vi "TestFGV.vi"() -> ()   [LabVIEW 2015]
uses:
  TypeDef/RoomsActionEnum.ctl
panel:
  out "Flag Out 4":bool[](array[boolean])
  out "Flag Out 3":bool[](array[boolean])
  out "Flag Out 2":bool[](array[boolean])
  out "Flag Out":bool[](array[boolean])
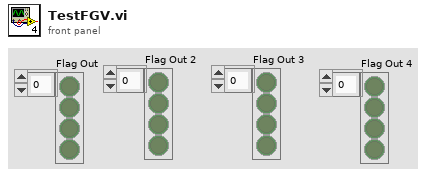
[diagram p1: front panel]
types:
  T1 = typedef "RoomsActionEnum.ctl" = enum16{"Init", "Add Room", "Remove Room", "Read Room", "Read Flag", "Read Flag State", "Write Flag State", "Read Flag Color", "Write Flag Color", "Read Bed Vacant", "Write Bed Vacant", "Read Personnel", "Add Personnel", "Remove Personnel", "Read Requests", "Add Request", "Remove Request", "Read Beacon ID", "Write Beacon ID", "Write Bed URL", "Read Bed URL"}
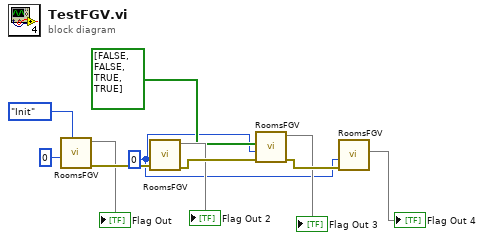
[diagram p0: block diagram]
diagram:
  w1 = 0 ("Room")
  n1 = call "RoomsFGV.vi"("Actions"=RoomsActionEnum."Init", "Data In"=0 ("Room")) -> ("error out"=w12:errorcluster, 2:→"Flag Out")  [unwired: 7 in, 1 out]
  n2 = call "RoomsFGV.vi"("error in (no error)"=w12, "Data In"=w1) -> ("error out"=w11:errorcluster, 2:→"Flag Out 2", "Actions"=w8:T1)  [unwired: 6 in, 1 out]
  n3 = call "RoomsFGV.vi"("error in (no error)"=w11, "Data In"=w1, "Room"=bool[] [FALSE, FALSE, TRUE, TRUE] ("Flag In")) -> ("error out"=w10:errorcluster, 2:→"Flag Out 3", "Actions"=w3:T1)  [unwired: 5 in, 1 out]
  n4 = call "RoomsFGV.vi"("error in (no error)"=w10, "Data In"=w1) -> (2:→"Flag Out 4", "Actions"=w4:T1)  [unwired: 6 in, 2 out]
